vi "OpenCLV Manual.vi"   [LabVIEW 2012]
uses:
  <vilib>/Platform/browser.llb/Open URL in Default Browser (path).vi
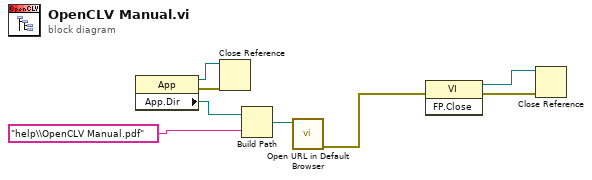
[diagram p0: block diagram]
diagram:
  n1 = property class="App"() -> (reference out=w5:refnum<vi>, error out=w6:errorcluster, "App.Dir"=w4:path)  [unwired: 2 in]
  n2 = Close Reference(reference=w5, error in (no error)=w6) -> ()  [unwired: 1 out]
  n3 = Build Path(base path=w4, name or relative path="help\\OpenCLV Manual.pdf") -> (appended path=w7:path)
  n4 = call-poly <vilib>:"Open URL in Default Browser.vi"("path"=w7) -> ("error out"=w1:errorcluster)  [unwired: 5 in, 1 out]
  n5 = invoke class="VI" method="FP.Close"(error in=w1) -> (reference out=w2:refnum<vi>, error out=w3:errorcluster)  [unwired: 2 in, 1 out]
  n6 = Close Reference(reference=w2, error in (no error)=w3) -> ()  [unwired: 1 out]
